vi "Create_scan_testing_array.vi"() -> (12 "Total frames":dbl, 13 "conflict":bool, 14 "Int. Scan Array 1":dbl[](array[numeric]), 15 "Int. Scan Array 2":dbl[](array[numeric]), 17 "Stop Value 1":dbl, 18 "Stop Value 2":dbl, 19 "Est. (t)":dbl caption="Est. Time (s)")   [LabVIEW 2015]
uses:
  MARS_Scan_Global_var.vi
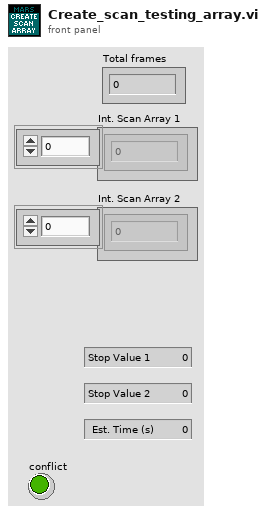
[diagram p1: front panel]
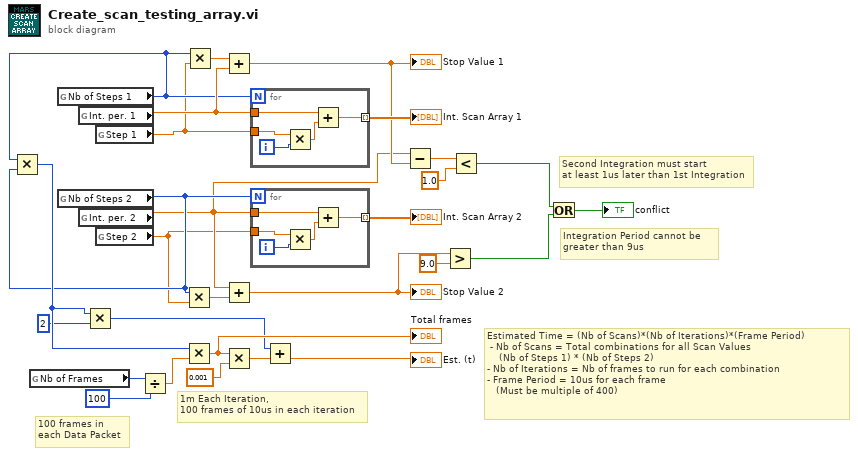
[diagram p0: block diagram]
diagram:
  # "100 frames in \neach Data Packet"
  # "Integration Period cannot be \ngreater than 9us"
  # "Second Integration must start \nat least 1us later than 1st Integration"
  # "Estimated Time = (Nb of Scans)*(Nb of Iterations)*(Frame Period)\n - Nb of Scans = Total combinations for all Scan Values\n    (Nb of Steps 1) * (Nb of Steps 2) \n- Nb of Iterations = Nb of frames to run for each combination\n- Frame Period = 10us for each frame \n   (Must be multiple of 400)"
  # "1m Each Iteration,\n100 frames of 10us in each iteration"
  n1 = global read "MARS_Scan_Global_var.vi" "Nb of Frames"() -> (w3:u32)
  n2 = global read "MARS_Scan_Global_var.vi" "Nb of Steps 1"() -> (w8:u16)
  n3 = global read "MARS_Scan_Global_var.vi" "Nb of Steps 2"() -> (w6:u16)
  n4 = Multiply(x=w8, y=w6) -> (x*y=w13:u16)
  n5 = global read "MARS_Scan_Global_var.vi" "Int. per. 1"() -> (w9:dbl)
  n6 = global read "MARS_Scan_Global_var.vi" "Int. per. 2"() -> (w5:dbl)
  n7 = Multiply(x=w13, y=u16 2) -> (x*y=w10:u16)
  n8 = global read "MARS_Scan_Global_var.vi" "Step 1"() -> (w7:dbl)
  n9 = global read "MARS_Scan_Global_var.vi" "Step 2"() -> (w4:dbl)
  n10 = Divide(x=w3, y=u32 100) -> (x/y=w1:dbl)
  n11 = Multiply(x=w6, y=w4) -> (x*y=w25:dbl)
  n12 = Multiply(x=w13, y=w1) -> (x*y=w15:dbl)
  "Total frames" <- w15
  n13 = Multiply(x=w8, y=w7) -> (x*y=w26:dbl)
  n14 = Add(x=w26, y=w9) -> (x+y=w23:dbl)
  "Stop Value 1" <- w23
  n15 = Add(x=w5, y=w25) -> (x+y=w20:dbl)
  "Stop Value 2" <- w20
  n16 = Multiply(x=w15, y=0.001) -> (x*y=w24:dbl)
  n17 = for {
    N: w8 -> [_]
    tunnel: w9 -> [w32]
    tunnel: [w30] -> w28 mode=indexing
    tunnel: w7 -> [w29]
    i -> [w33]
    n18 = Multiply(x=w29, y=w33) -> (x*y=w31:dbl)
    n19 = Add(x=w32, y=w31) -> (x+y=w30:dbl)
  }
  "Int. Scan Array 1" <- w28
  n20 = for {
    N: w6 -> [_]
    tunnel: w5 -> [w37]
    tunnel: [w35] -> w27 mode=indexing
    tunnel: w4 -> [w34]
    i -> [w38]
    n21 = Multiply(x=w34, y=w38) -> (x*y=w36:dbl)
    n22 = Add(x=w37, y=w36) -> (x+y=w35:dbl)
  }
  "Int. Scan Array 2" <- w27
  n23 = Add(x=w10, y=w24) -> (x+y=→"Est. (t)":dbl)
  n24 = Subtract(x=w5, y=w23) -> (x-y=w22:dbl)
  n25 = Greater?(x=w20, y=9.0) -> (0:w18:bool)
  n26 = Less?(x=w22, y=1.0) -> (x < y?=w17:bool)
  n27 = Or(x=w17, y=w18) -> (x .or. y?=→"conflict":bool)
